vi "auto sl.vi"() -> ()   [LabVIEW 2012, in "Mecanum Drive.lvrbt"]
uses:
  Mecanum Drive.lvrbt
  SubVIs/State_Typ.ctl
  <vilib>/NXT/HiTechnic/HiTechnic Controls/HiTechnic Port.ctl
  <vilib>/NXT/Block Support/NXT_InputPort.ctl
  SubVIs/auto_drive_TYP.ctl
  <vilib>/NXT/Hardware/Plugins/Tetrix DC Motor/TetrixDCMotorAddress.ctl
  <vilib>/NXT/Dual Mode Library/Display/drawNumber.vi
  <vilib>/NXT/NXTIO Xnodes/NXTIONodeSubVIs/TETRIX IO Check Battery.vi
  <vilib>/NXT/Dual Mode Library/Waits/Wait_Num(msec).vi
  <vilib>/NXT/NXTIO Xnodes/NXTIONodeSubVIs/TETRIX IO Reset Encoders.vi
  <vilib>/NXT/NXTIO Xnodes/NXTIONodeSubVIs/TETRIX IO Motor Status.vi
  <vilib>/NXT/NXTIO Xnodes/NXTIONodeSubVIs/TETRIX IO Stop DC Motors.vi
  <vilib>/NXT/Dual Mode Library/Sound/Tone.vi
  <vilib>/NXT/Dual Mode Library/Waits/Wait_Num.vi
  <vilib>/NXT/Subs/LVHSConnector.ctl
  <vilib>/NXT/NXTIO Xnodes/AddressXNode/NXTIOAddress.xnode
  <vilib>/NXT/NXTIO Xnodes/NXTIOXNode/NXTIO.xnode
  <vilib>/NXT/LegoClasses/BrickReference/BrickReference.lvclass
panel:
  out "Enabled":bool
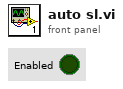
[diagram p1: front panel]
types:
  T1 = typedef "auto_drive_TYP.ctl" = cluster{"Left X":i8, "Left Y":i8, "Right X":i8, "Power (100)":i8, "Wait (ms)":u32, "Enc/Deg Target":i32, "Move Type":enum16{"Relative Degrees", "Wait", "Encoder"}}
  T2 = typedef "State_Typ.ctl" = enum16{"Stop", "Check for Position 3", "Check for Position 2", "Move", "Reset Enc", "Read Enc"}
  T3 = typedef "HiTechnic Port.ctl" = cluster{"Port":T4, "MUX Port":u8}
  T4 = typedef "NXT_InputPort.ctl" = u32
  T5 = typedef "TetrixDCMotorAddress.ctl" = i32
  T6 = typedef "LVHSConnector.ctl" = refnum<class "BrickReference.lvclass">
  T7 = cluster{"TetrixDCMotor":T5, "TetrixDCMotor 2":T5}
  T8 = cluster{"Direction (0-9)":i16, "Signal Strength (Array)":u8[]}
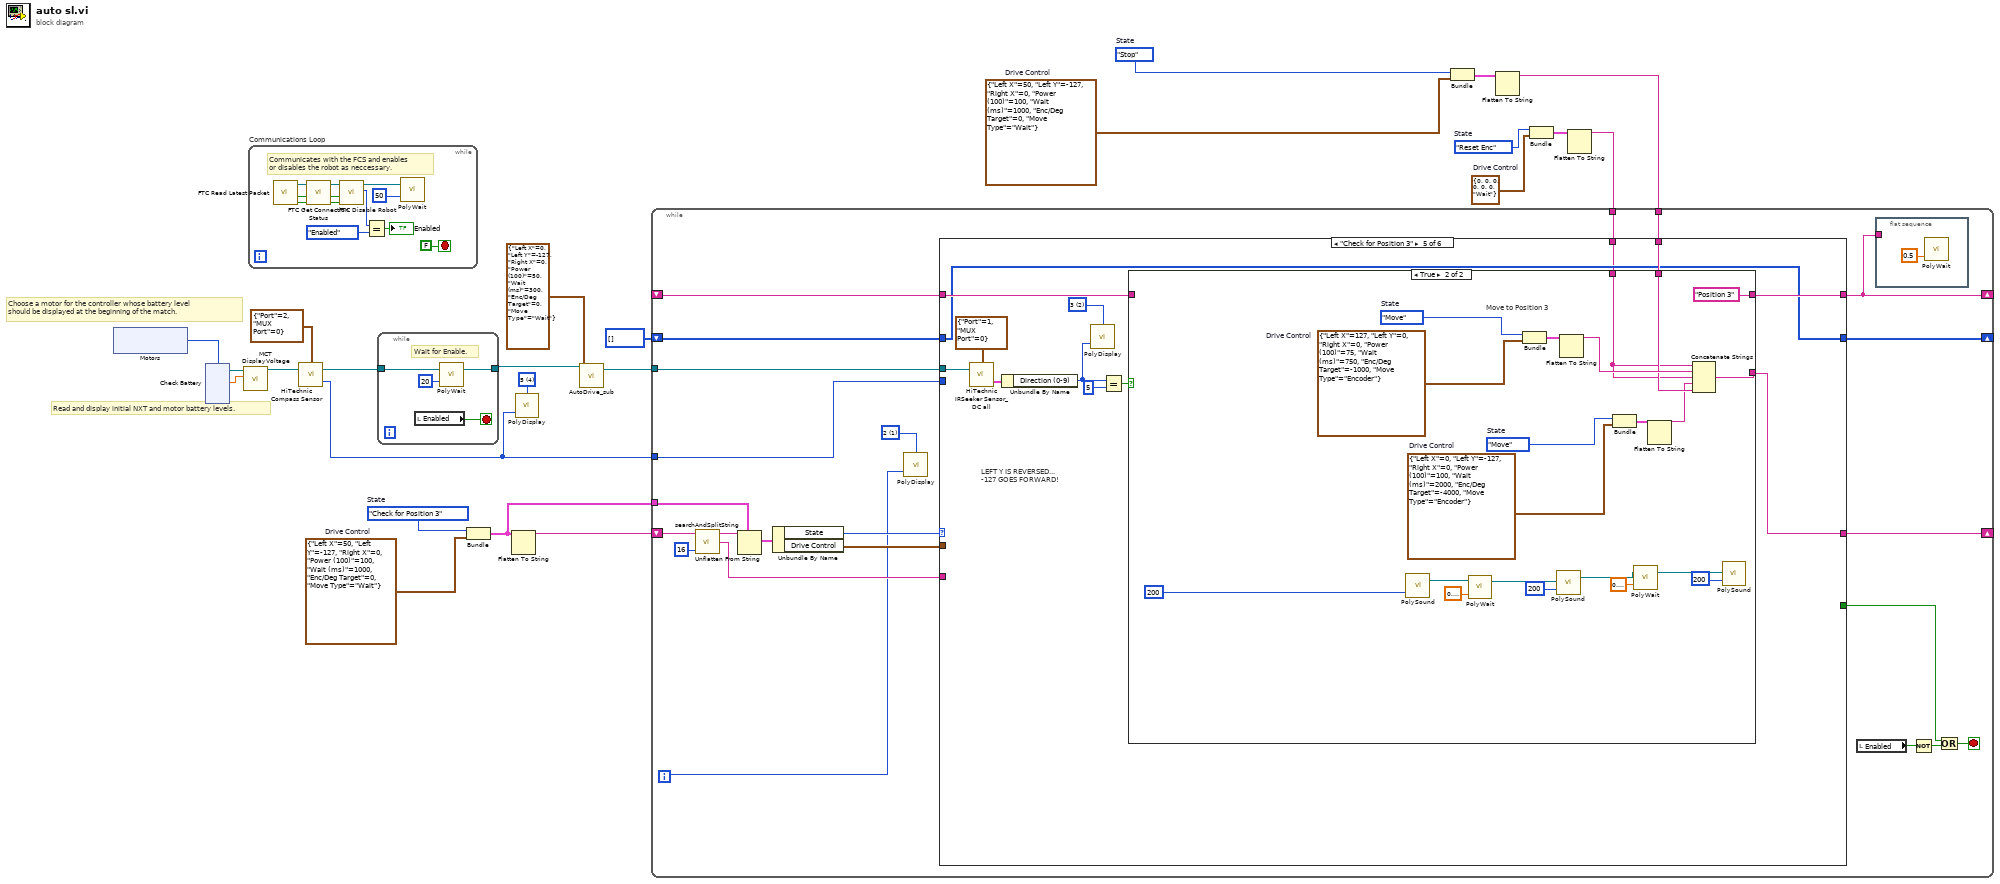
[diagram p0: block diagram]
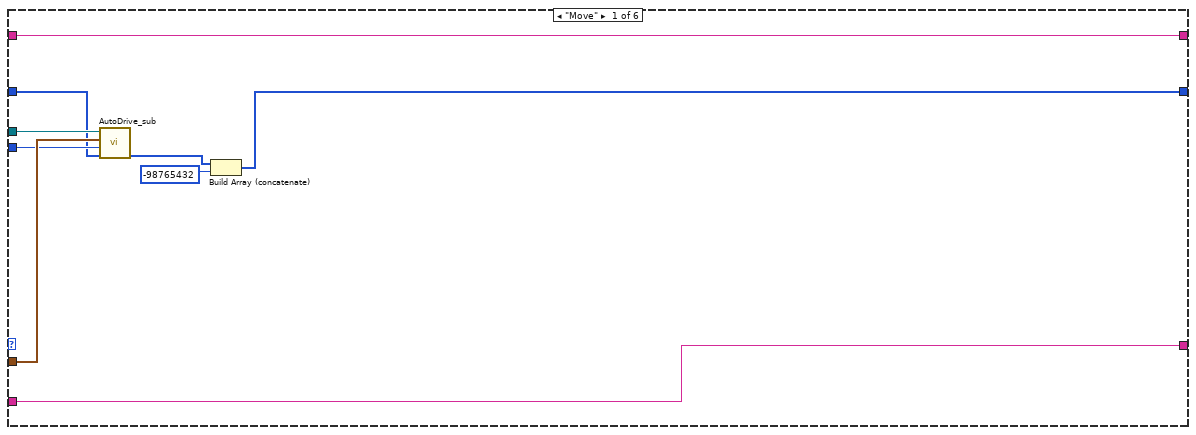
[diagram p2: hidden frame]
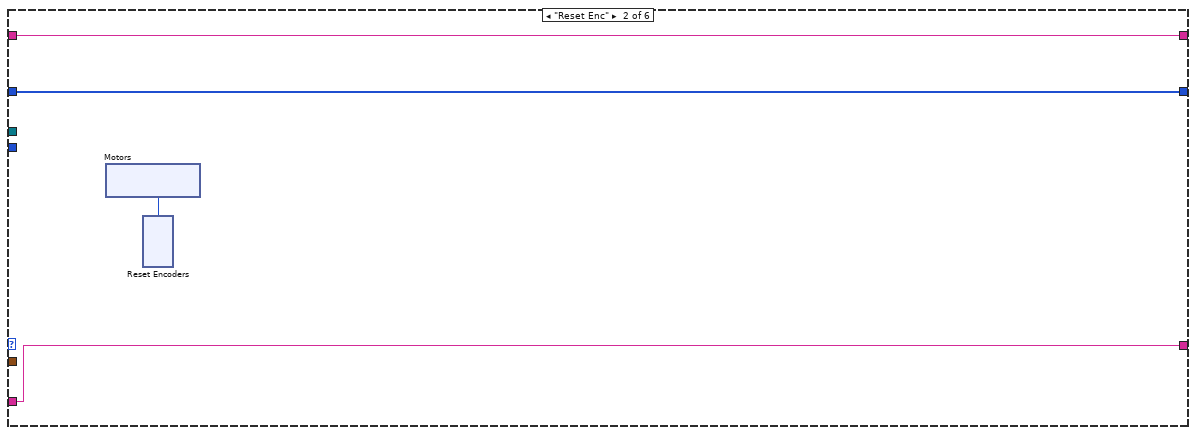
[diagram p3: hidden frame]
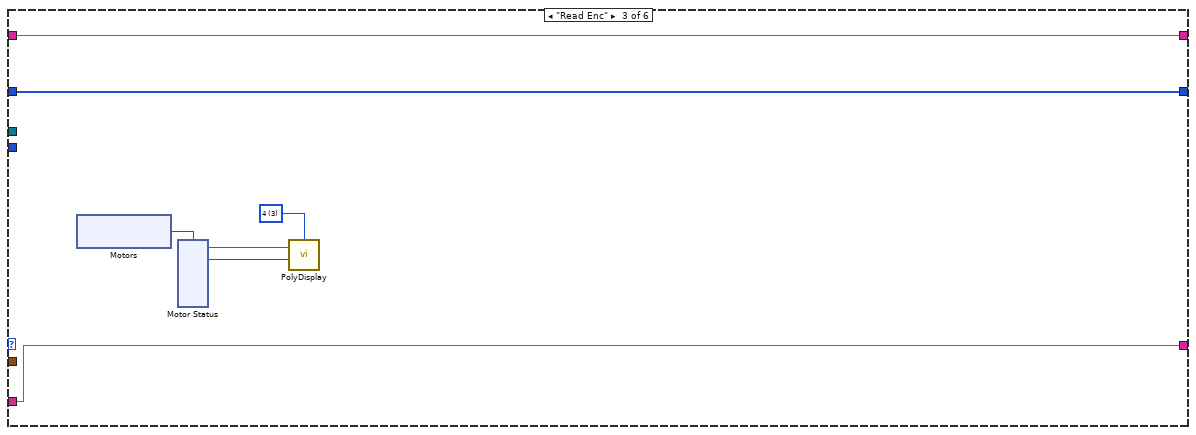
[diagram p4: hidden frame]
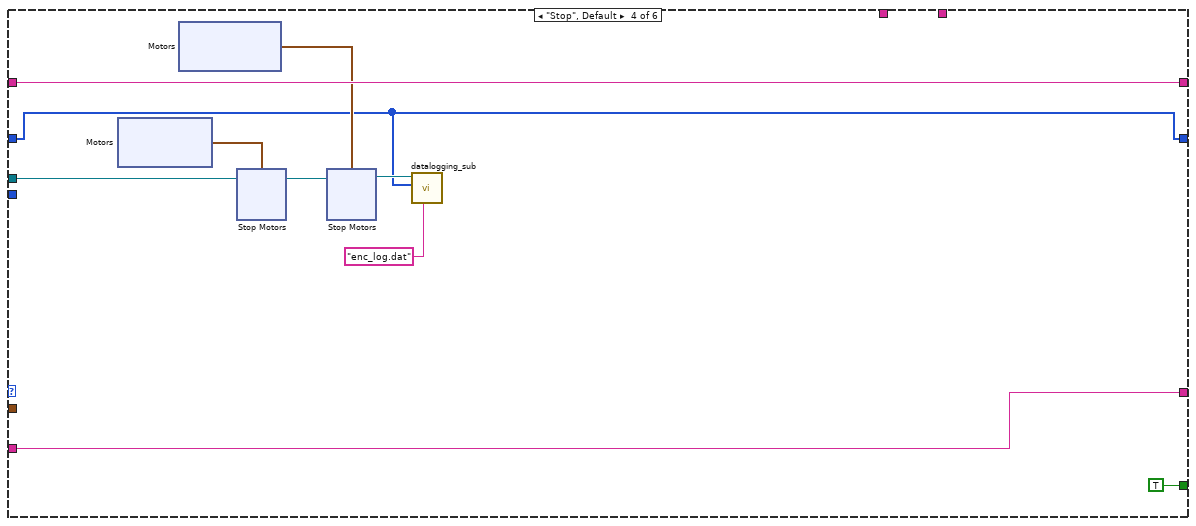
[diagram p5: hidden frame]
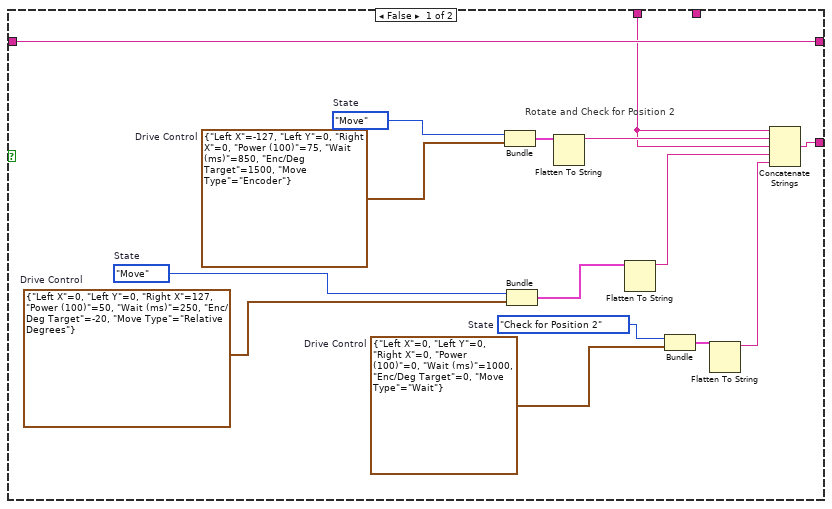
[diagram p6: hidden frame]
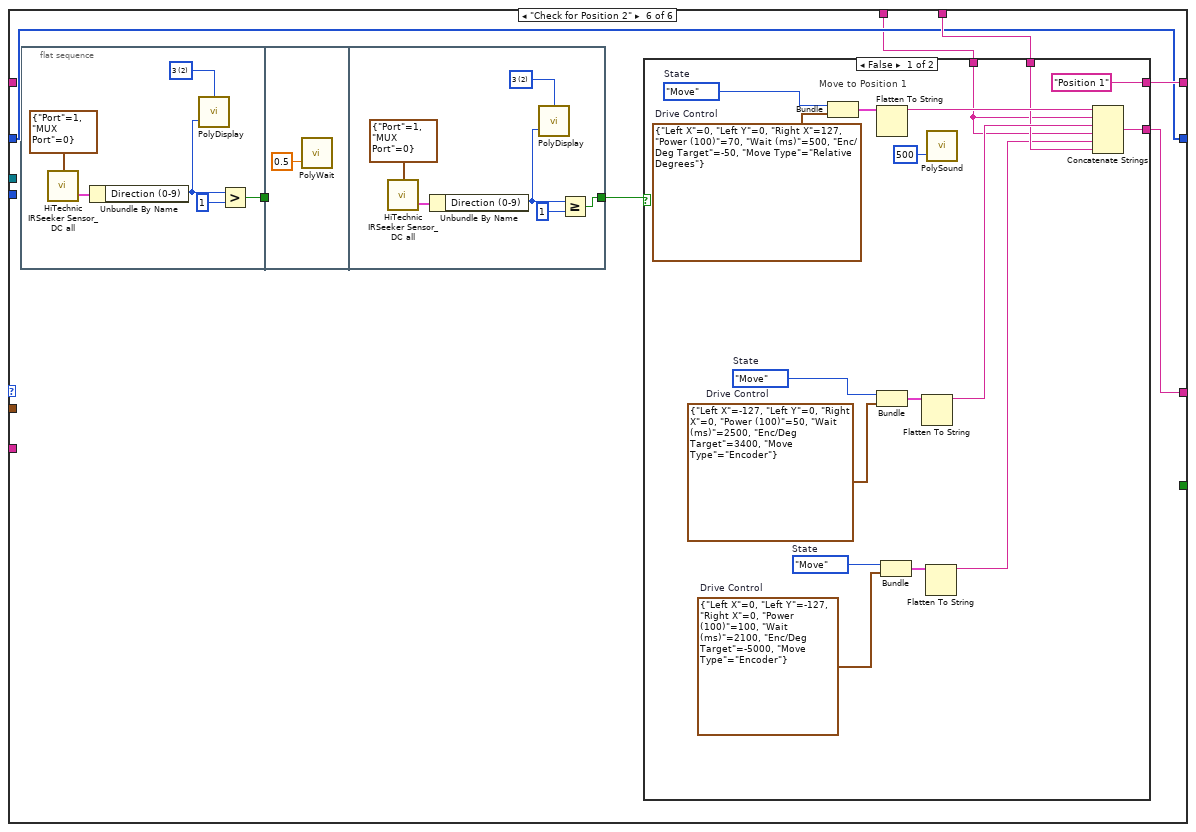
[diagram p7: hidden frame]
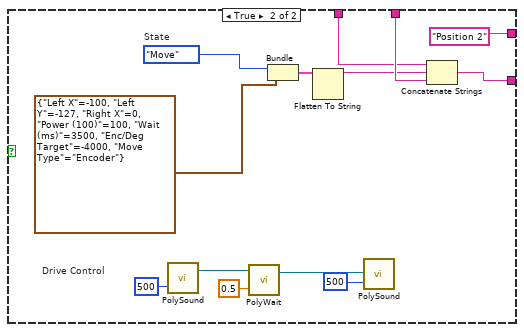
[diagram p8: hidden frame]
diagram:
  w1 = T1 {"Left X"=0, "Left Y"=0, "Right X"=0, "Power (100)"=0, "Wait (ms)"=0, "Enc/Deg Target"=0, "Move Type"=enum."Wait"}  # Drive Control
  w3 = State_Typ."Reset Enc"  # State
  w11 = T1 {"Left X"=50, "Left Y"=-127, "Right X"=0, "Power (100)"=100, "Wait (ms)"=1000, "Enc/Deg Target"=0, "Move Type"=enum."Wait"}  # Drive Control
  w12 = State_Typ."Stop"  # State
  w15 = i16 4 items=["1", "2", "3", "4", "5", "6", "7", "8", "9", "10", "11", "12"] ("Line")
  w24 = T1 {"Left X"=50, "Left Y"=-127, "Right X"=0, "Power (100)"=100, "Wait (ms)"=1000, "Enc/Deg Target"=0, "Move Type"=enum."Wait"}  # Drive Control
  w23 = State_Typ."Check for Position 3"  # State
  # "Read and display initial NXT and motor battery levels."
  # "Choose a motor for the controller whose battery level \nshould be displayed at the beginning of the match."
  n1 = xnode "Motors"() -> ("Motor"=w20:T5)
  n2 = xnode "Check Battery"("Motors"=w20) -> ("Voltage 1"=w21:sgl, "NXT/EV3"=w22:T6)  [unwired: 1 in]
  n3 = call <vilib>:"MCT DisplayVoltage.vi"("Motor Voltage"=w21, "NXT"=w22) -> ("NXT"=w16:T6)  [unwired: 9 in]
  n4 = while "Communications Loop" {
    stop <- FALSE stop-if-true
    # "Communicates with the FCS and enables \nor disables the robot as neccessary."
    n5 = call <vilib>:"FTC Read Latest Packet.vi"() -> ("Packet Received?"=w34:bool, "Stopped?"=w33:bool, "NXT"=w36:T6)  [unwired: 6 in, 3 out]
    n6 = call <vilib>:"FTC Get Connection Status.vi"("Packet Received?"=w34, "Stopped?"=w33, "NXT"=w36) -> ("Online?"=w25:bool, "Stopped?"=w26:bool, "NXT"=w35:T6)  [unwired: 5 in]
    n7 = call <vilib>:"FTC Disable Robot.vi"("Online?"=w25, "Stopped?"=w26, "NXT"=w35) -> ("Enabled?"=w29:enum16{"Disabled", "Enabled"}, "NXT"=w31:T6)  [unwired: 3 in]
    n8 = Equal?(x=w29, y=enum16{"Disabled", "Enabled"}."Enabled") -> (x = y?=→"Enabled":bool)
    n9 = call-poly <vilib>:"PolyWait.vi"("Time (100 msec)"=u32 50 ("Time (msec)"), "NXT/EV3"=w31) -> ()  [unwired: 2 in, 1 out]
  }
  n10 = call <vilib>:"HiTechnic Compass Sensor.vi"("NXT/EV3"=w16, "Port/MUX"=T3 {"Port"=2, "MUX Port"=0}) -> ("Heading (degrees)"=w14:i16, "NXT/EV3"=w9:T6)  [unwired: 1 in]
  n11 = while {
    tunnel: [w38] -> w7
    tunnel: w9 -> [w37]
    stop <- w39 stop-if-true
    # "Wait for Enable."
    n12 = local read "Enabled"() -> (w39:bool)
    n13 = call-poly <vilib>:"PolyWait.vi"("Time (100 msec)"=u32 20 ("Time (msec)"), "NXT/EV3"=w37) -> ("NXT/EV3"=w38:T6)  [unwired: 2 in]
  }
  n14 = Bundle("State"=w23, "Drive Control"=w24) -> (w19:cluster{"State":T2, "Drive Control":T1})  [unwired: 1 in]
  n15 = Flatten To String(anything=w19) -> (data string=w18:string)  [unwired: 3 in, 2 out]
  n16 = call-poly <vilib>:"PolyDisplay.vi"("number"=w14, "Line"=w15) -> ()  [unwired: 2 in, 1 out]
  n17 = call "AutoDrive_sub.vi"("Drive Control"=T1 {"Left X"=0, "Left Y"=-127, "Right X"=0, "Power (100)"=50, "Wait (ms)"=300, "Enc/Deg Target"=0, "Move Type"=enum."Wait"}, "NXT/EV3"=w7) -> ("NXT/EV3 out"=w8:T6)  [unwired: 8 in, 1 out]
  n18 = Bundle("State"=w12, "Drive Control"=w11) -> (w13:cluster{"State":T2, "Drive Control":T1})  [unwired: 1 in]
  n19 = Flatten To String(anything=w13) -> (data string=w10:string)  [unwired: 3 in, 2 out]
  n20 = Bundle("State"=w3, "Drive Control"=w1) -> (w4:cluster{"State":T2, "Drive Control":T1})  [unwired: 1 in]
  n21 = Flatten To String(anything=w4) -> (data string=w2:string)  [unwired: 3 in, 2 out]
  n22 = while {
    tunnel: w8 -> [w63]
    shift-right: [w54] -> _
    shift-left: w18 -> [w52]
    tunnel: w19 -> [w55]
    shift-right: [w45] -> _
    shift-left: _ -> [w53]
    tunnel: w10 -> [w50]
    tunnel: w14 -> [w44]
    shift-right: [w43] -> _
    shift-left: i32[] [] -> [w42]
    tunnel: w2 -> [w41]
    i -> [w46]
    stop <- w62 stop-if-true
    w47 = i16 1 items=["1", "2", "3", "4", "5", "6", "7", "8", "9", "10", "11", "12"] ("Line")
    n23 = call <vilib>:"searchAndSplitString.vi"("offset (0)"=16 ("length (rest)"), "string"=w52) -> ("match + rest of string"=w51:string, "substring before match"=w57:string)  [unwired: 1 in, 1 out]
    n24 = Unflatten From String(type=w55, binary string=w57) -> (value=w56:cluster{"State":T2, "Drive Control":T1})  [unwired: 3 in, 2 out]
    n25 = Unbundle By Name(w56) -> ("State"=w48:T2, "Drive Control"=w58:T1)
    n26 = call-poly <vilib>:"PolyDisplay.vi"("number"=w46, "Line"=w47) -> ()  [unwired: 2 in, 1 out]
    n27 = case shown="\"Check for Position 3\"" w48 {
      tunnel: w63 -> [w73 _ _ w108 w131 _]
      tunnel: [_ _ _ TRUE _ _] -> w61
      tunnel: w58 -> [w72 _ _ _ _ _]
      tunnel: w51 -> [w71 w77 w89 w106 _ _]
      tunnel: [w71 w77 w89 w106 w127 w173] -> w54
      tunnel: [w70 w76 w88 w105 w130 w175] -> w45
      tunnel: w53 -> [w70 w76 w88 w105 w129 _]
      tunnel: w50 -> [_ _ _ _ w128 w174]
      tunnel: w44 -> [w69 _ _ _ _ _]
      tunnel: [w68 w74 w83 w100 w122 w171] -> w43
      tunnel: w42 -> [w66 w74 w83 w100 w122 w171]
      tunnel: w41 -> [_ _ _ _ w121 w170]
      frame "Move" {
        n28 = call "AutoDrive_sub.vi"("EncoderVals"=w66, "Target Heading (Degrees)"=w69, "Drive Control"=w72, "NXT/EV3"=w73) -> ("EncoderVals"=w65:i32[])  [unwired: 6 in, 1 out]
        n29 = Build Array (concatenate)(w65, -98765432 ("new element/subarray")) -> (w68:i32[])
      }
      frame "Reset Enc" {
        n30 = xnode "Motors"() -> ("Motor"=w75:T5)
        n31 = xnode "Reset Encoders"("Motors"=w75) -> ()  [unwired: 1 in, 1 out]
      }
      frame "Read Enc" {
        w85 = i16 3 items=["1", "2", "3", "4", "5", "6", "7", "8", "9", "10", "11", "12"] ("Line")
        n32 = xnode "Motors"() -> ("Motor"=w87:T5)
        n33 = xnode "Motor Status"("Motors"=w87) -> ("Position 1"=w86:i32, "NXT/EV3"=w84:T6)  [unwired: 1 in, 1 out]
        n34 = call-poly <vilib>:"PolyDisplay.vi"("number"=w86, "NXT/EV3"=w84, "Line"=w85) -> ()  [unwired: 1 in, 1 out]
      }
      frame "Stop", Default {
        n35 = xnode "Motors"() -> ("Motor"=w104:cluster{"TetrixDCMotor":T5, "TetrixDCMotor":T5})
        n36 = xnode "Motors"() -> ("Motor"=w103:cluster{"TetrixDCMotor":T5, "TetrixDCMotor":T5})
        n37 = xnode "Stop Motors"("Motors"=w104, "NXT/EV3"=w108) -> ("NXT/EV3"=w102:T6)
        n38 = xnode "Stop Motors"("Motors"=w103, "NXT/EV3"=w102) -> ("NXT/EV3"=w101:T6)
        n39 = call "datalogging_sub.vi"("Filename"="enc_log.dat", "Encoder Vals"=w100, "NXT/EV3 In"=w101) -> ()  [unwired: 8 in, 1 out]
      }
      frame "Check for Position 3" {
        w124 = i16 2 items=["1", "2", "3", "4", "5", "6", "7", "8", "9", "10", "11", "12"] ("Line")
        # "LEFT Y IS REVERSED...\n-127 GOES FORWARD!"
        n40 = call <vilib>:"HiTechnic IRSeeker Sensor_DC all.vi"("NXT/EV3"=w131, "Port/MUX"=T3 {"Port"=1, "MUX Port"=0}) -> ("All Info"=w133:T8)  [unwired: 1 in, 1 out]
        n41 = Unbundle By Name(w133) -> ("Direction (0-9)"=w125:i16)
        n42 = call-poly <vilib>:"PolyDisplay.vi"("number"=w125, "Line"=w124) -> ()  [unwired: 2 in, 1 out]
        n43 = Equal?(x=w125, y=i16 5) -> (x = y?=w123:bool)
        n44 = case shown="True" w123 {
          tunnel: [w143 w162] -> w127
          tunnel: [w142 "Position 3"] -> w130
          tunnel: w129 -> [w142 _]
          tunnel: w128 -> [_ w160]
          tunnel: w121 -> [w134 w149]
          frame False {
            w138 = T1 {"Left X"=0, "Left Y"=0, "Right X"=127, "Power (100)"=50, "Wait (ms)"=250, "Enc/Deg Target"=-20, "Move Type"=enum."Relative Degrees"}  # Drive Control
            w139 = State_Typ."Move"  # State
            w147 = T1 {"Left X"=0, "Left Y"=0, "Right X"=0, "Power (100)"=0, "Wait (ms)"=1000, "Enc/Deg Target"=0, "Move Type"=enum."Wait"}  # Drive Control
            w148 = State_Typ."Check for Position 2"  # State
            w141 = T1 {"Left X"=-127, "Left Y"=0, "Right X"=0, "Power (100)"=75, "Wait (ms)"=850, "Enc/Deg Target"=1500, "Move Type"=enum."Encoder"}  # Drive Control
            w144 = State_Typ."Move"  # State
            # "Rotate and Check for Position 2"
            n45 = Bundle("State"=w144, "Drive Control"=w141) -> (w145:cluster{"State":T2, "Drive Control":T1})  [unwired: 1 in]
            n46 = Bundle("State"=w139, "Drive Control"=w138) -> (w140:cluster{"State":T2, "Drive Control":T1})  [unwired: 1 in]
            n47 = Flatten To String(anything=w145) -> (data string=w135:string)  [unwired: 3 in, 2 out]
            n48 = Flatten To String(anything=w140) -> (data string=w137:string)  [unwired: 3 in, 2 out]
            n49 = Bundle("State"=w148, "Drive Control"=w147) -> (w146:cluster{"State":T2, "Drive Control":T1})  [unwired: 1 in]
            n50 = Flatten To String(anything=w146) -> (data string=w136:string)  [unwired: 3 in, 2 out]
            n51 = Concatenate Strings(w134, w135, w134, w137, w136) -> (w143:string)
          }
          frame True {
            w166 = T1 {"Left X"=0, "Left Y"=-127, "Right X"=0, "Power (100)"=100, "Wait (ms)"=2000, "Enc/Deg Target"=-4000, "Move Type"=enum."Encoder"}  # Drive Control
            w167 = State_Typ."Move"  # State
            w169 = T1 {"Left X"=127, "Left Y"=0, "Right X"=0, "Power (100)"=75, "Wait (ms)"=750, "Enc/Deg Target"=-1000, "Move Type"=enum."Encoder"}  # Drive Control
            w168 = State_Typ."Move"  # State
            # "Move to Position 3"
            n52 = call-poly <vilib>:"PolySound.vi"("Duration (500 ms)"=u16 200) -> ("NXT/EV3"=w156:T6)  [unwired: 3 in]
            n53 = call-poly <vilib>:"PolyWait.vi"("Time (1 sec)"=sgl 0.2, "NXT/EV3"=w156) -> ("NXT/EV3"=w155:T6)  [unwired: 2 in]
            n54 = Bundle("State"=w168, "Drive Control"=w169) -> (w165:cluster{"State":T2, "Drive Control":T1})  [unwired: 1 in]
            n55 = call-poly <vilib>:"PolySound.vi"("Duration (500 ms)"=u16 200, "NXT/EV3"=w155) -> ("NXT/EV3"=w152:T6)  [unwired: 2 in]
            n56 = Flatten To String(anything=w165) -> (data string=w163:string)  [unwired: 3 in, 2 out]
            n57 = Bundle("State"=w167, "Drive Control"=w166) -> (w164:cluster{"State":T2, "Drive Control":T1})  [unwired: 1 in]
            n58 = call-poly <vilib>:"PolyWait.vi"("Time (1 sec)"=sgl 0.2, "NXT/EV3"=w152) -> ("NXT/EV3"=w151:T6)  [unwired: 2 in]
            n59 = Flatten To String(anything=w164) -> (data string=w150:string)  [unwired: 3 in, 2 out]
            n60 = Concatenate Strings(w149, w163, w149, w150, w160) -> (w162:string)
            n61 = call-poly <vilib>:"PolySound.vi"("Duration (500 ms)"=u16 200, "NXT/EV3"=w151) -> ()  [unwired: 2 in, 1 out]
          }
        }
      }
      frame "Check for Position 2" {
        n62 = flat-sequence {
          tunnel: [w180] -> w172
          tunnel: w172 -> [_]
          tunnel: [w184] -> w176
          frame #0 {
            w177 = i16 2 items=["1", "2", "3", "4", "5", "6", "7", "8", "9", "10", "11", "12"] ("Line")
            n63 = call <vilib>:"HiTechnic IRSeeker Sensor_DC all.vi"("Port/MUX"=T3 {"Port"=1, "MUX Port"=0}) -> ("All Info"=w182:T8)  [unwired: 2 in, 1 out]
            n64 = Unbundle By Name(w182) -> ("Direction (0-9)"=w178:i16)
            n65 = call-poly <vilib>:"PolyDisplay.vi"("number"=w178, "Line"=w177) -> ()  [unwired: 2 in, 1 out]
            n66 = Greater?(x=w178, y=i16 1) -> (0:w180:bool)
          }
          frame #1 {
            n67 = call-poly <vilib>:"PolyWait.vi"("Time (1 sec)"=sgl 0.5) -> ()  [unwired: 3 in, 1 out]
          }
          frame #2 {
            w189 = i16 2 items=["1", "2", "3", "4", "5", "6", "7", "8", "9", "10", "11", "12"] ("Line")
            n68 = call <vilib>:"HiTechnic IRSeeker Sensor_DC all.vi"("Port/MUX"=T3 {"Port"=1, "MUX Port"=0}) -> ("All Info"=w185:T8)  [unwired: 2 in, 1 out]
            n69 = Unbundle By Name(w185) -> ("Direction (0-9)"=w188:i16)
            n70 = call-poly <vilib>:"PolyDisplay.vi"("number"=w188, "Line"=w189) -> ()  [unwired: 2 in, 1 out]
            n71 = Greater Or Equal?(x=w188, y=i16 1) -> (x >= y?=w184:bool)
          }
        }
        n72 = case shown="False" w176 {
          tunnel: [w203 w216] -> w173
          tunnel: ["Position 1" "Position 2"] -> w175
          tunnel: w174 -> [w195 w209]
          tunnel: w170 -> [w190 w207]
          frame False {
            w193 = T1 {"Left X"=0, "Left Y"=-127, "Right X"=0, "Power (100)"=100, "Wait (ms)"=2100, "Enc/Deg Target"=-5000, "Move Type"=enum."Encoder"}  # Drive Control
            w194 = State_Typ."Move"  # State
            w201 = T1 {"Left X"=-127, "Left Y"=0, "Right X"=0, "Power (100)"=50, "Wait (ms)"=2500, "Enc/Deg Target"=3400, "Move Type"=enum."Encoder"}  # Drive Control
            w202 = State_Typ."Move"  # State
            w205 = T1 {"Left X"=0, "Left Y"=0, "Right X"=127, "Power (100)"=70, "Wait (ms)"=500, "Enc/Deg Target"=-50, "Move Type"=enum."Relative Degrees"}  # Drive Control
            w206 = State_Typ."Move"  # State
            # "Move to Position 1"
            n73 = Bundle("State"=w206, "Drive Control"=w205) -> (w204:cluster{"State":T2, "Drive Control":T1})  [unwired: 1 in]
            n74 = Flatten To String(anything=w204) -> (data string=w197:string)  [unwired: 3 in, 2 out]
            n75 = Bundle("State"=w202, "Drive Control"=w201) -> (w200:cluster{"State":T2, "Drive Control":T1})  [unwired: 1 in]
            n76 = Bundle("State"=w194, "Drive Control"=w193) -> (w192:cluster{"State":T2, "Drive Control":T1})  [unwired: 1 in]
            n77 = Flatten To String(anything=w200) -> (data string=w199:string)  [unwired: 3 in, 2 out]
            n78 = Flatten To String(anything=w192) -> (data string=w191:string)  [unwired: 3 in, 2 out]
            n79 = call-poly <vilib>:"PolySound.vi"("Duration (500 ms)"=u16 500) -> ()  [unwired: 3 in, 1 out]
            n80 = Concatenate Strings(w197, w190, w199, w190, w191, w195) -> (w203:string)
          }
          frame True {
            w218 = T1 {"Left X"=-100, "Left Y"=-127, "Right X"=0, "Power (100)"=100, "Wait (ms)"=3500, "Enc/Deg Target"=-4000, "Move Type"=enum."Encoder"}  # Drive Control
            w217 = State_Typ."Move"  # State
            n81 = call-poly <vilib>:"PolySound.vi"("Duration (500 ms)"=u16 500) -> ("NXT/EV3"=w211:T6)  [unwired: 3 in]
            n82 = call-poly <vilib>:"PolyWait.vi"("Time (1 sec)"=sgl 0.5, "NXT/EV3"=w211) -> ("NXT/EV3"=w210:T6)  [unwired: 2 in]
            n83 = Bundle("State"=w217, "Drive Control"=w218) -> (w219:cluster{"State":T2, "Drive Control":T1})  [unwired: 1 in]
            n84 = Flatten To String(anything=w219) -> (data string=w208:string)  [unwired: 3 in, 2 out]
            n85 = call-poly <vilib>:"PolySound.vi"("Duration (500 ms)"=u16 500, "NXT/EV3"=w210) -> ()  [unwired: 2 in, 1 out]
            n86 = Concatenate Strings(w207, w208, w209) -> (w216:string)
          }
        }
      }
    }
    n87 = local read "Enabled"() -> (w60:bool)
    n88 = flat-sequence {
      tunnel: w45 -> [_]
      frame #0 {
        n89 = call-poly <vilib>:"PolyWait.vi"("Time (1 sec)"=sgl 0.5) -> ()  [unwired: 3 in, 1 out]
      }
    }
    n90 = Not(x=w60) -> (.not. x?=w49:bool)
    n91 = Or(x=w61, y=w49) -> (x .or. y?=w62:bool)
  }
